vi "2Voice.Button_FrameCheck.vi"(7 "timeout (10sec)":u32=2000 caption="超时（10秒）", 8 "error in (no error)":errorcluster caption="错误输入（无错误）", 10 "Frame CMD":T1(ring), 11 "FrameReader Port":refnum<visa-resource-name> caption="VISA资源名称") -> (0 "错误输出":errorcluster, 1 "写入命令":u8[](array[numeric]) format="%02x", 2 "读取缓冲区":string, 3 "OK?":bool)   [LabVIEW 2012, in "Lib_UEL.ATE.lvlib" / "Lib_2Voice.lvlib"]
uses:
  <vilib>/Instr/_visa.llb/VISA Configure Serial Port (Instr).vi
  Lib_2Voice.lvlib
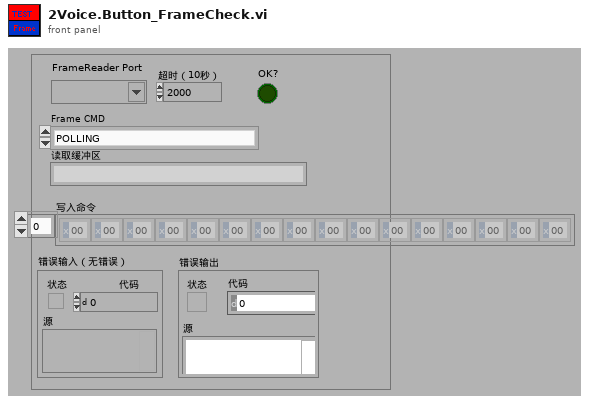
[diagram p1: front panel]
types:
  T1 = enum16{"POLLING", "CHIAMATA", "TEST_DRIVER", "ENTER_TEST_MODE", "CHIAMATA4AudioSetting", "CHIAMATA.FF", "POLLING.FF", "TEST(For BTWIN)"}
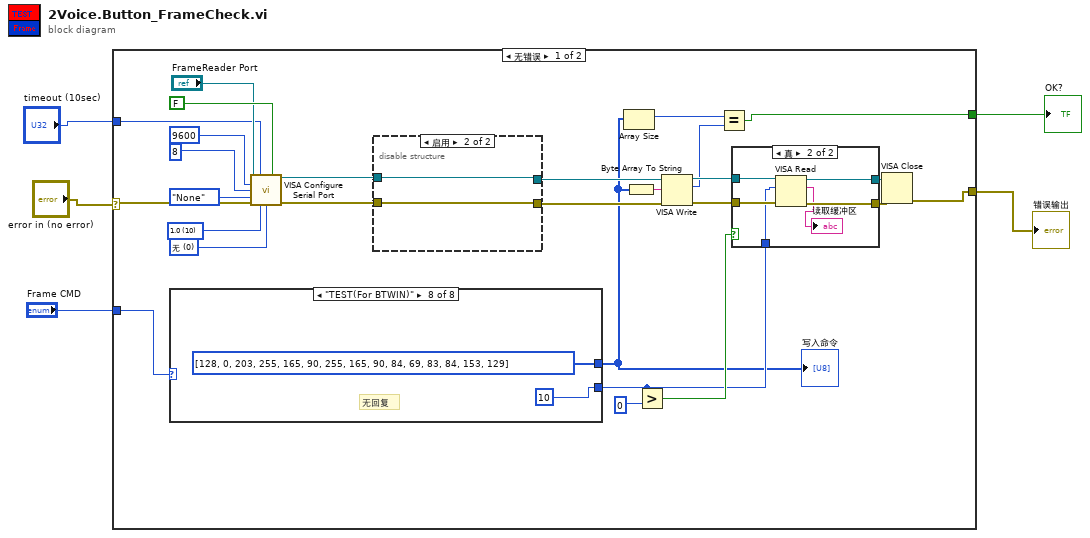
[diagram p0: block diagram]
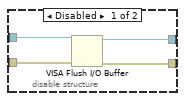
[diagram p2: hidden frame]
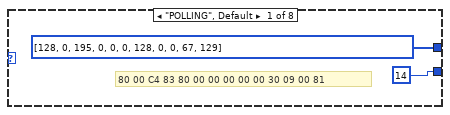
[diagram p4: hidden frame]
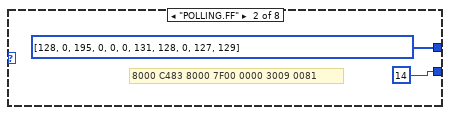
[diagram p5: hidden frame]
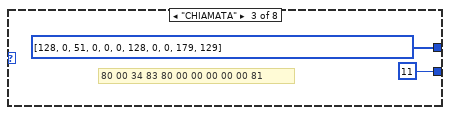
[diagram p6: hidden frame]
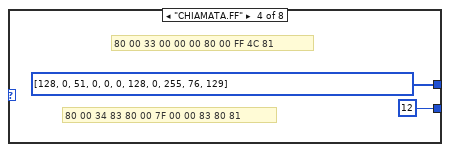
[diagram p7: hidden frame]
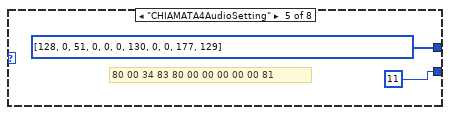
[diagram p8: hidden frame]
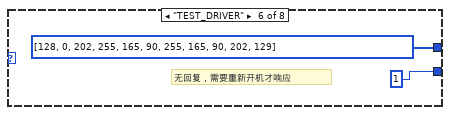
[diagram p9: hidden frame]
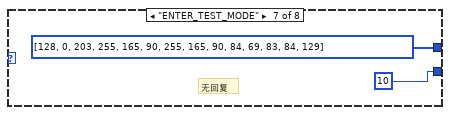
[diagram p10: hidden frame]
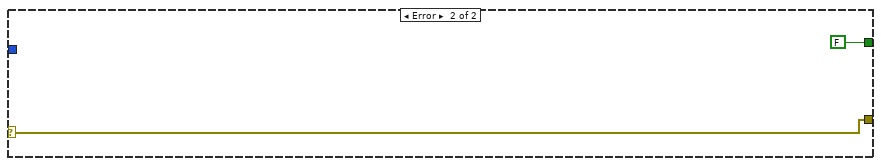
[diagram p11: hidden frame]
diagram:
  n1 = case shown="无错误" "error in (no error)" {
    selector: "error in (no error)" -> [w24 w64]
    tunnel: "Frame CMD" -> [w25 _]
    tunnel: [w16 w64] -> w3
    tunnel: "timeout (10sec)" -> [w14 _]
    tunnel: [w7 FALSE] -> w1
    frame No Error {
      w32 = u16 0 items=["无", "XON/XOFF", "RTS/CTS", "XON/XOFF & RTS/CTS", "DTR/DSR", "XON/XOFF & DTR/DSR"] ("flow control (0:none)")
      w31 = u16 10 items=["1.0"=10, "1.5"=15, "2.0"=20] ("stop bits (10: 1 bit)")
      n2 = case shown="\"TEST(For BTWIN)\"" w25 {
        tunnel: [u8[] [128, 0, 195, 0, 0, 0, 128, 0, 0, 67, 129] ("无符号字节数组") u8[] [128, 0, 195, 0, 0, 0, 131, 128, 0, 127, 129] ("无符号字节数组") u8[] [128, 0, 51, 0, 0, 0, 128, 0, 0, 179, 129] ("无符号字节数组") u8[] [128, 0, 51, 0, 0, 0, 128, 0, 255, 76, 129] ("无符号字节数组") u8[] [128, 0, 51, 0, 0, 0, 130, 0, 0, 177, 129] ("无符号字节数组") u8[] [128, 0, 202, 255, 165, 90, 255, 165, 90, 202, 129] ("无符号字节数组") u8[] [128, 0, 203, 255, 165, 90, 255, 165, 90, 84, 69, 83, 84, 129] ("无符号字节数组") u8[] [128, 0, 203, 255, 165, 90, 255, 165, 90, 84, 69, 83, 84, 153, 129] ("无符号字节数组")] -> w6
        tunnel: [14 ("y") 14 ("y") 11 12 11 1 ("y") 10 ("y") 10 ("y")] -> w19
        frame "POLLING", Default {
          # "80 00 C4 83 80 00 00 00 00 00 30 09 00 81"
        }
        frame "POLLING.FF" {
          # "8000 C483 8000 7F00 0000 3009 0081"
        }
        frame "CHIAMATA" {
          # "80 00 34 83 80 00 00 00 00 00 81"
        }
        frame "CHIAMATA.FF" {
          # "80 00 34 83 80 00 7F 00 00 83 80 81"
          # "80 00 33 00 00 00 80 00 FF 4C 81"
        }
        frame "CHIAMATA4AudioSetting" {
          # "80 00 34 83 80 00 00 00 00 00 81"
        }
        frame "TEST_DRIVER" {
          # "无回复，需要重新开机才响应"
        }
        frame "ENTER_TEST_MODE" {
          # "无回复"
        }
        frame "TEST(For BTWIN)" {
          # "无回复"
        }
      }
      "写入命令" <- w6
      n3 = call-poly "VISA Configure Serial Port"("VISA resource name"="FrameReader Port", "timeout (10sec)"=w14, "Enable Termination\nChar (T)"=FALSE ("Disable Termination\nChar (T)"), "baud rate (9600)"=u32 9600, "data bits (8)"=u16 8, "parity (0:none)"=enum16{"None", "Odd", "Even", "Mark", "Space"}."None", "error in (no error)"=w24, "stop bits (10: 1 bit)"=w31, "flow control (0:none)"=w32) -> ("VISA resource name out"=w13:refnum<visa-resource-name>, "error out"=w12:errorcluster)  [unwired: 5 in]
      n4 = disable-structure shown="启用" {
        disable-tunnel: w13 -> [w36 w38]
        disable-tunnel: w12 -> [w35 w37]
        disable-tunnel: [w34 w38] -> w11
        disable-tunnel: [w33 w37] -> w10
        frame Disabled {
          n5 = VISA Flush I/O Buffer(VISA resource name=w36, error in (no error)=w35) -> (VISA resource name out=w34:refnum<visa-resource-name>, error out=w33:errorcluster)  [unwired: 1 in]
        }
        frame Enabled {
        }
      }
      n6 = Array Size(array=w6) -> (size(s)=w9:i32)
      n7 = Byte Array To String(unsigned byte array=w6) -> (string=w23:string)
      n8 = Greater?(x=w19, y=0) -> (0:w20:bool)
      n9 = VISA Write(VISA resource name=w11, write buffer=w23, error in (no error)=w10) -> (VISA resource name out=w21:refnum<visa-resource-name>, return count=w8:u32, error out=w22:errorcluster)
      n10 = Equal?(x=w9, y=w8) -> (x = y?=w7:bool)
      n11 = case shown="真" w20 {
        tunnel: w22 -> [w39 w46]
        tunnel: w21 -> [w40 w45]
        tunnel: w19 -> [_ w44]
        tunnel: [w40 w43] -> w18
        tunnel: [w39 w42] -> w17
        frame False {
        }
        frame True {
          n12 = VISA Read(VISA resource name=w45, byte count=w44, error in (no error)=w46) -> (VISA resource name out=w43:refnum<visa-resource-name>, read buffer=→"读取缓冲区":string, error out=w42:errorcluster)  [unwired: 1 out]
        }
      }
      n13 = VISA Close(VISA resource name=w18, error in (no error)=w17) -> (error out=w16:errorcluster)
    }
    frame Error {
    }
  }
  "错误输出" <- w3
  "OK?" <- w1
